vi "Main.vi"(11 "Module Admin":refnum<class "Delacor_lib_QMH_Module Admin.lvclass">) -> ()   [LabVIEW 2019, in "Acquisition.lvlib"]
doc: "This template is based off of the Queued Message Handler design pattern and the Queued Message Handler project template that ships with LabVIEW.\n\nThe main difference is that the queue is private to this module and communication between modules is performed via Broadcast and Request events.\n\nRequest events are wrapped in public API methods and are handled in the Event Handling Loop (EHL) of this VI. Any module can register for Broadcast events sent by this module. The EHL generates messages based on user interface actions.\n\nThe Message Handling Loop (MHL) processes messages generated by the EHL, or by other messages. The messages are string values, so new messages can be added easily to the Message Cases case structure in the MHL. Each message cluster can also provide an optional value for Message Data, which is a variant that can be converted to whatever message-specific data is required.\n_____\nBased on Delacor QMH Project Template 4.0.0.47.\n_____\nBased on Delacor QMH Project Template 5.0.0.82."
uses:
  Acquisition.lvlib
  <vilib>/Delacor/Delacor QMH/Libraries/Module Admin_class/Delacor_lib_QMH_Module Admin.lvclass
  Module Data--cluster.ctl
  Stop Argument--cluster.ctl
  <vilib>/Delacor/Delacor QMH/Libraries/Message Queue_class/Delacor_lib_QMH_Message Queue.lvclass/Delacor_lib_QMH_Message Queue.ctl
  <vilib>/Delacor/Delacor QMH/Libraries/Module Admin_class/Delacor_lib_QMH_Module Admin.lvclass/Delacor_lib_QMH_Module Admin.ctl
  Start Acquiring Argument--cluster.ctl
  Start Acquiring (Reply Payload)--cluster.ctl
  Stop Acquiring Argument--cluster.ctl
  Settings Editor/Update Application Settings (Reply Payload)--cluster.ctl
  Settings Editor/Settings--cluster.ctl
  <vilib>/Utility/miscctls.llb/LVPointTypeDef.ctl
  <vilib>/Delacor/Delacor QMH/Libraries/Message Queue_class/Delacor_lib_QMH_Enqueue Message (Single).vi
  <vilib>/Delacor/Delacor QMH/Libraries/Module Admin_class/Delacor_lib_QMH_Get External Launch.vi
  <vilib>/Utility/error.llb/Error Cluster From Error Code.vi
  <vilib>/ErrorRing/Error Ring.xnode
  <vilib>/Delacor/Delacor QMH/Libraries/Message Queue_class/Delacor_lib_QMH_Message Queue.lvclass
  Settings Editor/Settings Editor.lvlib
  Logger/Logger.lvlib
panel:
  out "Settings":T1={"Analog Input Channel"="", "Max Value"=0.0, "Min Value"=-5.0}
  out "Graph Data":waveform(dbl)[](array[waveform])
  out "error out":errorcluster
  # "This is a headless module. Show its panel to confirm that the Settings are updated correctly and other debugging tasks. Use the Settings Editor to change the settings for this module."
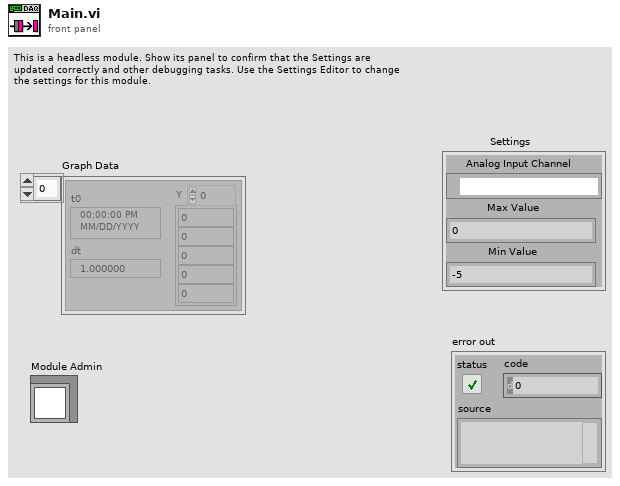
[diagram p1: front panel]
types:
  T1 = typedef "Acquisition.lvlib/Module Data--cluster.ctl" = cluster{"Analog Input Channel":refnum<k21>, "Max Value":dbl, "Min Value":dbl}
  T2 = typedef "Settings Editor.lvlib/Broadcast Events--cluster.ctl" = cluster{"Module Did Init":refnum<user-event>, "Status Updated":refnum<user-event>, "Error Reported":refnum<user-event>, "Module Did Stop":refnum<user-event>, "Update Module Execution Status":refnum<user-event>, "Application Settings Updated":refnum<user-event>}
  T3 = typedef "Acquisition.lvlib/Request Events--cluster.ctl" = cluster{"Stop Module":refnum<user-event>, "Show Panel":refnum<user-event>, "Hide Panel":refnum<user-event>, "Get Module Execution Status":refnum<user-event>, "Show Diagram":refnum<user-event>, "Stop Acquiring":refnum<user-event>, "Wakeup Helper Loop":refnum<user-event>, "Change Settings":refnum<user-event>, "Calibrate DAQ":refnum<user-event>, "Start Acquiring":refnum<user-event>}
  T4 = enum32{"invalid lock state", "Not Locked", "Locked (No Password)", "Password-protected"}
  T5 = typedef "Acquisition.lvlib/Stop Argument--cluster.ctl" = cluster{"Origin":string, "Exit via Stop Module Req?":bool, "Wait for Module to stop?":bool}
  T6 = typedef "Acquisition.lvlib/Start Acquiring Argument--cluster.ctl" = cluster{"Wait Notifier":refnum<notifier>, "wait for reply":bool}
  T7 = typedef "Acquisition.lvlib/Stop Acquiring Argument--cluster.ctl" = cluster{"Boolean":bool}
  T8 = typedef "Settings Editor.lvlib/Update Application Settings (Reply Payload)--cluster.ctl" = cluster{"Settings":T9, "Update Settings_error":errorcluster}
  T9 = typedef "Settings Editor.lvlib/Settings--cluster.ctl" = cluster{"Log File Base Path":path, "Analog Input Channel":refnum<k21>, "Max Value":dbl, "Min Value":dbl}
  T10 = typedef "LVPointTypeDef.ctl" = cluster{"Horizontal":i16, "Vertical":i16}
  T11 = enum32{"Invalid", "Standard", "Closed", "Hidden", "Minimized", "Maximized"}
  T12 = typedef "Acquisition.lvlib/Start Acquiring (Reply Payload)--cluster.ctl" = cluster{"HW ID":string, "Start Acquiring_error":errorcluster}
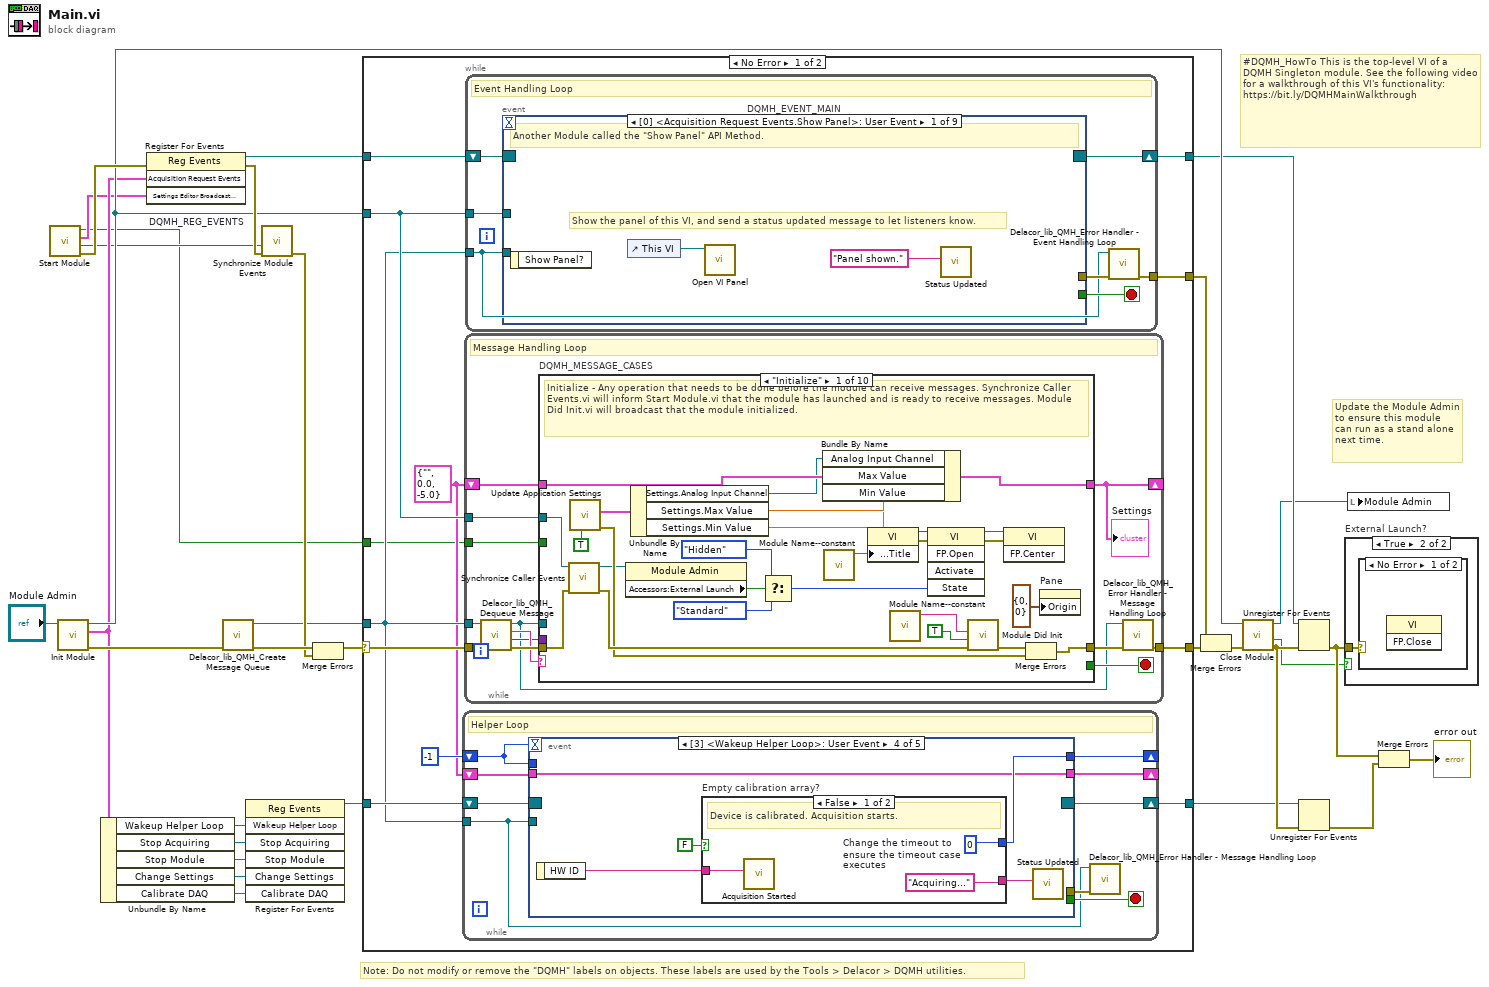
[diagram p0: block diagram]
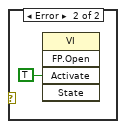
[diagram p3: hidden frame]
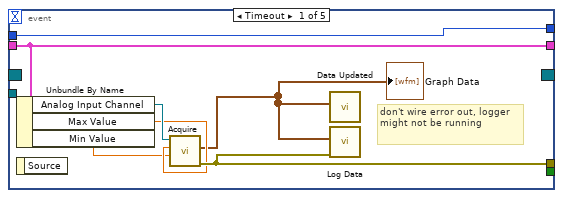
[diagram p4: hidden frame]
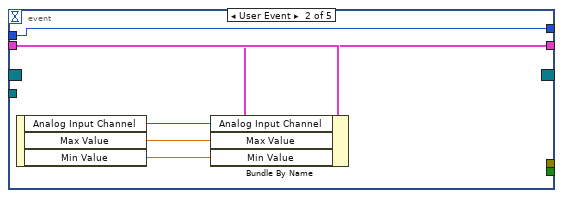
[diagram p5: hidden frame]
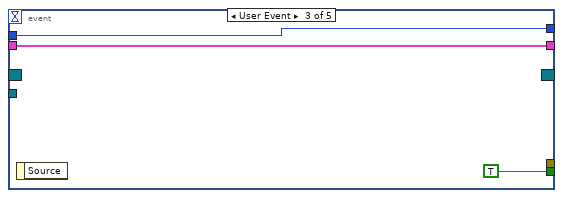
[diagram p6: hidden frame]
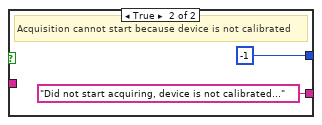
[diagram p7: hidden frame]
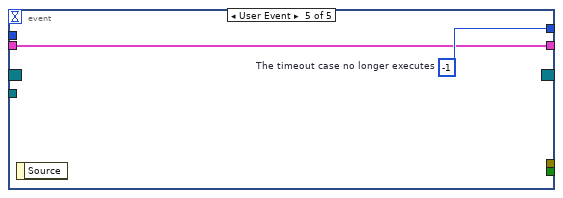
[diagram p8: hidden frame]
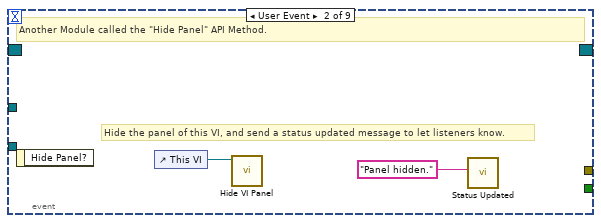
[diagram p9: hidden frame]
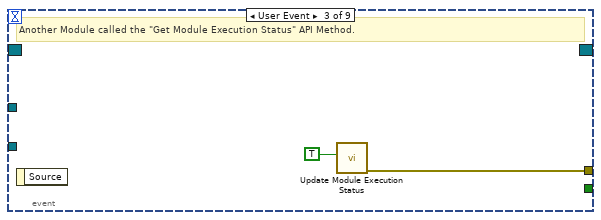
[diagram p10: hidden frame]
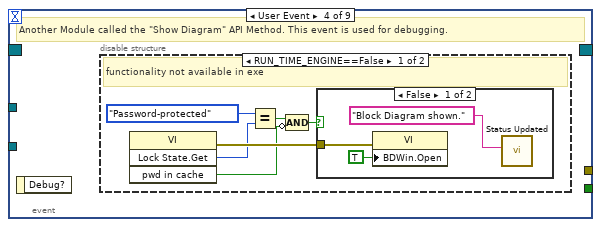
[diagram p11: hidden frame]
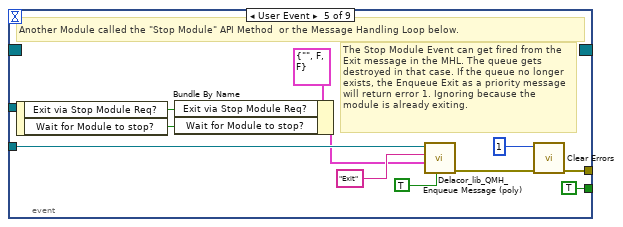
[diagram p14: hidden frame]
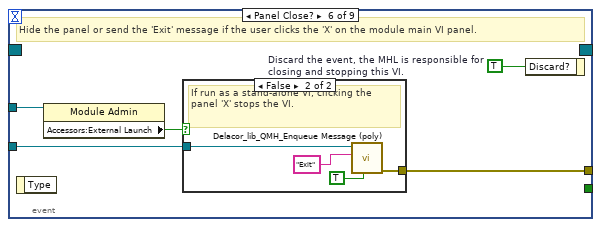
[diagram p15: hidden frame]
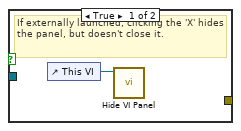
[diagram p16: hidden frame]
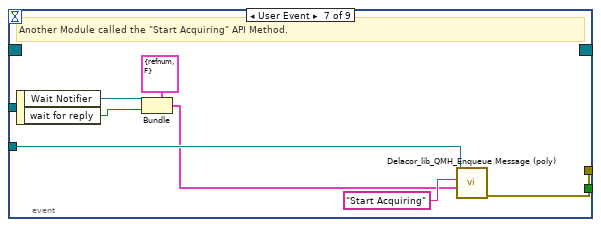
[diagram p17: hidden frame]
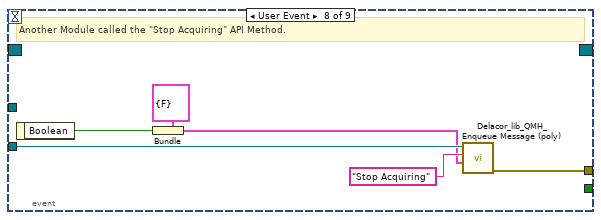
[diagram p18: hidden frame]
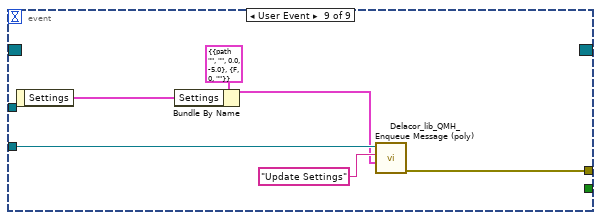
[diagram p19: hidden frame]
diagram:
  # "#DQMH_HowTo This is the top-level VI of a DQMH Singleton module. See the following video for a walkthrough of this VI's functionality: https://bit.ly/DQMHMainWalkthrough"
  # "Note: Do not modify or remove the \"DQMH\" labels on objects. These labels are used by the Tools > Delacor > DQMH utilities."
  # "Update the Module Admin to ensure this module can run as a stand alone next time."
  n1 = call "Start Module.vi"() -> ("error out"=w24:errorcluster, "Wait for Event Sync?"=w5:bool, "Settings Editor Broadcast Events"=w6:T2, "Module Was Already Running?"=w1:bool)  [unwired: 8 in]
  n2 = call "Init Module.vi"("Singleton Module Admin in"="Module Admin") -> ("error out"=w30:errorcluster, "Acquisition Request Events"=w11:T3, "Singleton Module Admin out"=w18:refnum<class "Delacor_lib_QMH_Module Admin.lvclass">)  [unwired: 8 in]
  n3 = Unbundle By Name(w11) -> ("Wakeup Helper Loop"=w7:refnum<user-event>, "Stop Acquiring"=w10:refnum<user-event>, "Stop Module"=w9:refnum<user-event>, "Change Settings"=w4:refnum<user-event>, "Calibrate DAQ"=w3:refnum<user-event>)
  n4 = register-events "DQMH_REG_EVENTS"(error in=w24, w11, w6) -> (reference out=w16:refnum<event-registration>, error out=w23:errorcluster)  [unwired: 1 in]
  n5 = call <vilib>:"Delacor_lib_QMH_Create Message Queue.vi"("error in"=w30) -> ("error out"=w26:errorcluster, "Message Queue"=w15:refnum<class "Delacor_lib_QMH_Message Queue.lvclass">)  [unwired: 9 in]
  n6 = register-events(w7, w10, w9, w4, w3) -> (reference out=w8:refnum<event-registration>)  [unwired: 2 in, 1 out]
  n7 = call "Synchronize Module Events.vi"("error in (no error)"=w23, "Wait for Event Sync?"=w5) -> ("error out"=w22:errorcluster)  [unwired: 9 in]
  n8 = Merge Errors(w26, w22) -> (w25:errorcluster)
  n9 = case shown="No Error" w25 {
    selector: w25 -> [w41 w279]
    tunnel: [w43 w278] -> w31
    tunnel: [w40 w287] -> w17
    tunnel: w16 -> [w39 w287]
    tunnel: w15 -> [w35 w280]
    tunnel: [w42 _] -> w29
    tunnel: w18 -> [w38 w283]
    tunnel: w8 -> [w36 w282]
    tunnel: [w33 w282] -> w2
    tunnel: w1 -> [w32 w281]
    frame No Error {
      w34 = T1 {"Analog Input Channel"="", "Max Value"=0.0, "Min Value"=-5.0} ("Data Cluster")
      n10 = while {
        shift-right: [w51] -> _
        shift-left: -1 -> [w50]
        tunnel: w35 -> [w47]
        shift-right: [w46] -> _
        shift-left: w34 -> [w45]
        shift-right: [w44] -> w33
        shift-left: w36 -> [w49]
        stop <- w48 stop-if-true
        # "Helper Loop"
        n11 = event shown="[3] <Wakeup Helper Loop>: User Event" {
          selector: w49 -> [_ _ _ _ _]
          dyn-events: [_ _ _ _ _] -> w44
          timeout: w50 -> [_ _ _ _ _]
          tunnel: [w58 w65 w68 w73 w80] -> w51
          tunnel: w50 -> [w58 w65 w68 _ _]
          tunnel: [_ _ TRUE _ _] -> w48
          tunnel: w47 -> [_ _ _ _ _]
          tunnel: [w59 _ _ _ _] -> w52
          tunnel: [w57 w63 w66 w70 w79] -> w46
          tunnel: w45 -> [w57 w64 w66 w70 w79]
          event Timeout {
            # "don't wire error out, logger might not be running"
            n12 = Unbundle By Name(w57) -> ("Analog Input Channel"=w56:refnum<k21>, "Max Value"=w55:dbl, "Min Value"=w54:dbl)
            n13 = event-data() -> ()  [unwired: 1 in, 1 out]
            n14 = call "Acquire.vi"("Min Value"=w54, "Max Value"=w55, "Refnum in"=w56) -> ("error out"=w59:errorcluster, "Graph Data"=w53:waveform(dbl)[])  [unwired: 7 in]
            "Graph Data" <- w53
            n15 = call "Data Updated.vi"("Graph Data"=w53) -> ()  [unwired: 10 in, 1 out]
            n16 = call "Log Data.vi"("error in (no error)"=w59, "Waveforms"=w53) -> ()  [unwired: 9 in, 1 out]
          }
          event User Event {
            n17 = event-data() -> ("Analog Input Channel"=w60:refnum<k21>, "Max Value"=w62:dbl, "Min Value"=w61:dbl)  [unwired: 1 in]
            n18 = Bundle By Name(cluster=w64, "Analog Input Channel"=w60, "Max Value"=w62, "Min Value"=w61) -> (w63:T1)
          }
          event User Event {
            n19 = event-data() -> ()  [unwired: 1 in, 1 out]
          }
          event User Event {
            n20 = event-data() -> ("HW ID"=w71:string)  [unwired: 1 in]
            n21 = case "Empty calibration array?" shown="False" FALSE {
              tunnel: ["Acquiring..." ("Status") "Did not start acquiring, device is not calibrated..." ("Status")] -> w72
              tunnel: [w75 -1] -> w73
              tunnel: w71 -> [w76 _]
              frame False {
                w75 = 0  # Change the timeout to ensure the timeout case executes
                # "Device is calibrated. Acquisition starts."
                n22 = call "Acquisition Started.vi"("HW ID"=w76) -> ()  [unwired: 10 in, 1 out]
              }
              frame True {
                # "Acquisition cannot start because device is not calibrated"
              }
            }
            n23 = call "Status Updated.vi"("Status"=w72) -> ()  [unwired: 10 in, 1 out]
          }
          event User Event {
            w80 = -1  # The timeout case no longer executes
            n24 = event-data() -> ()  [unwired: 1 in, 1 out]
          }
        }
        n25 = call-dynamic "Delacor_lib_QMH_Error Handler - Message Handling Loop.vi"("error in"=w52, "Message Queue in"=w47) -> ()  [unwired: 8 in, 2 out]
      }
      n26 = while {
        tunnel: w35 -> [w147]
        shift-right: [w143] -> _
        shift-left: w34 -> [w151]
        tunnel: w41 -> [w154]
        tunnel: [w152] -> w43
        tunnel: w38 -> [w145]
        tunnel: w32 -> [w144]
        stop <- w150 stop-if-true
        # "Message Handling Loop"
        n27 = call-dynamic "Delacor_lib_QMH_Dequeue Message.vi"("error in"=w154, "Message Queue in"=w147) -> ("error out"=w153:errorcluster, "Message Data"=w148:variant, "Message"=w149:string, "Message Queue out"=w146:refnum<class "Delacor_lib_QMH_Message Queue.lvclass">)  [unwired: 6 in]
        n28 = case "DQMH_MESSAGE_CASES" shown="\"Initialize\"" w149 {
          selector: w149 -> [_ _ _ _ _ _ _ _ _ w265]
          tunnel: w146 -> [_ _ _ _ _ _ _ w230 w254 _]
          tunnel: w153 -> [w179 w183 w196 w210 w221 w224 w226 w237 w261 w268]
          tunnel: [w176 w183 w194 w208 w213 w223 w226 w233 w258 w269] -> w155
          tunnel: w151 -> [w166 w182 w184 w205 w218 w222 w225 w232 w246 w266]
          tunnel: [w161 w182 w192 w205 w218 w222 w225 w232 w246 w266] -> w143
          tunnel: [_ _ _ _ _ _ _ _ w253 _] -> w150
          tunnel: w148 -> [_ _ w191 w207 w219 _ _ w231 w252 _]
          tunnel: w145 -> [w167 _ _ _ _ _ _ w229 w247 _]
          tunnel: w144 -> [_ _ _ _ _ _ _ _ w244 _]
          frame "Initialize" {
            # "Initialize - Any operation that needs to be done before the module can receive messages. Synchronize Caller Events.vi will inform Start Module.vi that the module has launched and is ready to receive messages. Module Did Init.vi will broadcast that the module initialized."
            n29 = call "Synchronize Caller Events.vi"("error in (no error)"=w179, "Singleton Module Admin in"=w167) -> ("error out"=w178:errorcluster, "Singleton Module Admin out"=w163:refnum<class "Delacor_lib_QMH_Module Admin.lvclass">)  [unwired: 8 in]
            n30 = call "Update Application Settings.vi"("wait for reply (T)"=TRUE) -> ("error out"=w175:errorcluster, "Reply Payload"=w160:T8)  [unwired: 8 in, 1 out]
            n31 = property class="Module Admin"(reference=w163) -> ("Accessors:External Launch"=w171:bool)  [unwired: 1 in, 2 out]
            n32 = Unbundle By Name(w160) -> ("Settings.Analog Input Channel"=w156:refnum<k21>, "Settings.Max Value"=w159:dbl, "Settings.Min Value"=w158:dbl)
            n33 = Select(t=T11."Hidden" ("State"), s=w171, f=T11."Standard" ("State")) -> (s? t:f=w168:T11)
            n34 = Bundle By Name(cluster=w166, "Analog Input Channel"=w156, "Max Value"=w159, "Min Value"=w158) -> (w161:T1)
            n35 = call "Module Name--constant.vi"() -> ("Module Name"=w174:string)  [unwired: 11 in]
            n36 = property class="VI"("Front Panel.Title"=w174) -> (reference out=w173:refnum<vi>, error out=w181:errorcluster)  [unwired: 2 in]
            n37 = call "Module Name--constant.vi"() -> ("Module Name"=w164:string)  [unwired: 11 in]
            n38 = invoke class="VI" method="FP.Open"(reference=w173, error in=w181, "State"=w168) -> (reference out=w172:refnum<vi>, error out=w180:errorcluster)  [unwired: 2 in, 3 out]
            n39 = call "Module Did Init.vi"("error in (no error)"=w178, "Initialized?"=TRUE, "Origin"=w164) -> ("error out"=w177:errorcluster)  [unwired: 8 in]
            n40 = invoke class="VI" method="FP.Center"(reference=w172, error in=w180) -> ()  [unwired: 1 in, 3 out]
            n41 = Merge Errors(w177, w175) -> (w176:errorcluster)
            n42 = property on="Pane" class="Pane"("Origin"=T10 {"Horizontal"=0, "Vertical"=0}) -> ()  [unwired: 2 in, 2 out]
          }
          frame "--- Module Specific ---" {
            # "Separator -- The following cases handle messages specific to this Module."
          }
          frame "Start Acquiring" {
            # "Requests Acquisition Module to start acquiring."
            n43 = Variant To Data(error in=w196, type=T6 {"Wait Notifier"=refnum, "wait for reply"=FALSE} ("Start Acquisition Argument"), Variant=w191) -> (data=w189:T6, error out=w193:errorcluster)
            n44 = in-place {
              in-place-border: [w202] -> w195
              in-place-border: w193 -> [w201]
              in-place-border: [w197] -> w185
              n45 = in-place-cluster #1(w184) -> ("Analog Input Channel"=w198:refnum<k21>)
              n46 = call "Initialize Hardware References.vi"("error in (no error)"=w201, "HW Refnum in"=w198) -> ("error out"=w200:errorcluster, "HW Refnum out"=w199:string)  [unwired: 8 in]
              n47 = call "Configure Hardware.vi"("error in (no error)"=w200, "HW Refnum in"=w199) -> ("error out"=w202:errorcluster, "HW Refnum out"=w197:string)  [unwired: 8 in]
              n48 = in-place-cluster #1("Analog Input Channel"=w197) -> (w192:T1)
            }
            n49 = Bundle By Name(cluster=T12 {"HW ID"="", "Start Acquiring_error"={"status"=FALSE, "code"=0, "source"=""}} ("Start Acquisition (Reply Payload)"), "HW ID"=w185, "Start Acquiring_error"=w195) -> (w187:T12)
            n50 = Unbundle By Name(w189) -> ("Wait Notifier"=w188:refnum<notifier>)
            n51 = call "Wakeup Helper Loop.vi"("error in (no error)"=w195, "HW ID"=w185) -> ("error out"=w194:errorcluster)  [unwired: 9 in]
            n52 = Send Notification(notification=w187, notifier=w188) -> ()  [unwired: 1 in, 2 out]
          }
          frame "Stop Acquiring" {
            # "Requests the Acquisition Module to stop acquiring"
            n53 = Variant To Data(error in=w210, type=T7 {"Boolean"=FALSE} ("Stop Acquiring Argument"), Variant=w207) -> (error out=w209:errorcluster)  [unwired: 1 out]
            n54 = Unbundle By Name(w205) -> ("Analog Input Channel"=w204:refnum<k21>)
            n55 = call "Stop Acquisition.vi"("error in (no error)"=w209, "HW Refnum"=w204) -> ("error out"=w208:errorcluster)  [unwired: 9 in]
            n56 = call "Acquisition Stopped.vi"("error in (no error)"=w208) -> ()  [unwired: 10 in, 1 out]
            n57 = call "Status Updated.vi"("error in (no error)"=w208, "Status"="Acquisition Stopped") -> ()  [unwired: 9 in, 1 out]
          }
          frame "Update Settings" {
            # "Send the Change Settings event to the helper loop."
            # "The Settings Editor broadcasted that the settings have changed."
            n58 = Variant To Data(error in=w221, type=T8 {"Settings"={"Log File Base Path"=path "", "Analog Input Channel"="", "Max Value"=0.0, "Min Value"=-5.0}, "Update Settings_error"={"status"=FALSE, "code"=0, "source"=""}} ("Settings Updated Argument"), Variant=w219) -> (data=w216:T8, error out=w220:errorcluster)
            n59 = Unbundle By Name(w216) -> ("Settings.Analog Input Channel"=w211:refnum<k21>, "Settings.Max Value"=w215:dbl, "Settings.Min Value"=w214:dbl)
            n60 = call "Change Settings.vi"("error in (no error)"=w220, "Min Value"=w214, "Max Value"=w215, "Analog Input Channel"=w211) -> ("error out"=w213:errorcluster)  [unwired: 7 in]
            n61 = call "Status Updated.vi"("error in (no error)"=w213, "Status"="Settings Updated") -> ()  [unwired: 9 in, 1 out]
          }
          frame "---Copy This Frame---" {
            # "Duplicate this frame when creating new messages.  Change this comment in the duplicated frame to describe this message."
            n62 = Merge Errors(w224) -> (w223:errorcluster)
          }
          frame "--- Exit and Error Handling---" {
            # "Separator - The following cases handle errors and exit messages."
          }
          frame "Error" {
            # "Error - Check the error message data and respond accordingly. This message is sent by the \"Error Handler\" VIs at the end of each loop in this application."
            n63 = property class="Module Admin"(reference=w229) -> ("Accessors:External Launch"=w228:bool)  [unwired: 1 in, 2 out]
            n64 = Variant To Data(error in=w237, type=errorcluster {"status"=FALSE, "code"=0, "source"=""} ("error constant"), Variant=w231) -> (data=w238:errorcluster, error out=w235:errorcluster)
            n65 = call "Module Name--constant.vi"() -> ("Module Name"=w227:string)  [unwired: 11 in]
            n66 = call "Error Reported.vi"("Additional Information"=w227, "Error"=w238) -> ()  [unwired: 9 in, 1 out]
            n67 = case shown="False" w228 {
              tunnel: [w243 _] -> w234
              tunnel: w230 -> [w241 _]
              tunnel: w238 -> [w242 _]
              frame False {
                # "If the module is running standalone, then pop up an error dialog and call the \"Exit\" message."
                n68 = call <vilib>:"Simple Error Handler.vi"("error in (no error)"=w242) -> ()  [unwired: 4 in, 5 out]
                n69 = call-poly <vilib>:"Delacor_lib_QMH_Enqueue Message (poly).vi"("Priority Message? (F)"=TRUE, "Message"="Exit", "Message Queue in"=w241) -> ("error out"=w243:errorcluster)  [unwired: 7 in, 1 out]
              }
              frame True {
                # "If the module was launched externally, calling the Error Reported broadcast VI is the only action performed by the \"Error\" message. The module's caller can then process the error appropriately."
              }
            }
            n70 = Merge Errors(w235, w234) -> (w233:errorcluster)
            n71 = local write "error out"(w233) -> ()
          }
          frame "Exit" {
            w251 = 91  # 91: not all Exit messages will have an argument
            w253 = TRUE  # Stop the VI
            # "Release the message queue reference"
            # "Exit - Exit the application."
            n72 = Variant To Data(error in=w261, type=T5 {"Origin"="", "Exit via Stop Module Req?"=FALSE, "Wait for Module to stop?"=FALSE} ("Stop Argument"), Variant=w252) -> (data=w249:T5, error out=w257:errorcluster)
            n73 = call <vilib>:"Clear Errors.vi"("error in (no error)"=w257, "specific error code to clear (0: all)"=w251) -> ("error out"=w260:errorcluster)  [unwired: 4 in, 1 out]
            n74 = Unbundle By Name(w246) -> ("Analog Input Channel"=w245:refnum<k21>)
            n75 = control-ref of="This VI"() -> (w248:refnum<vi>)
            n76 = call "Handle Exit.vi"("Stop Argument"=w249, "Admin in"=w247, "VI reference"=w248) -> ("error out"=w256:errorcluster)  [unwired: 7 in, 1 out]
            n77 = call "Close Hardware References.vi"("HW Refnum in"=w245) -> ("error out"=w255:errorcluster)  [unwired: 9 in, 1 out]
            n78 = call-dynamic "Delacor_lib_QMH_Release Message Queue.vi"("error in"=w260, "Message Queue"=w254) -> ("error out"=w259:errorcluster)  [unwired: 9 in]
            n79 = case "Settings Editor was\nalready running?" shown="False" w244 {
              frame False {
                n80 = call "Module Name--constant.vi"() -> ("Module Name"=w263:string)  [unwired: 11 in]
                n81 = call "Stop Module.vi"("Wait for Module to Stop? (F)"=TRUE, "Origin"=w263) -> ()  [unwired: 9 in, 1 out]
              }
              frame True {
                # "Another Module is\nin charge of stopping Settings Editor"
              }
            }
            n82 = Merge Errors(w259, w256, w255) -> (w258:errorcluster)
          }
          frame Default {
            # "'Default' case only runs if there is a message that isn't defined in any of the other cases.  Output a programming error."
            n83 = call "Module Name--constant.vi"() -> ("Module Name"=w264:string)  [unwired: 11 in]
            n84 = xnode "Error Ring"("parameter 0"=w265, "parameter 1"=w264) -> ("error out"=w267:errorcluster)
            n85 = Merge Errors(w268, w267) -> (w269:errorcluster)
          }
        }
        "Settings" <- w143
        n86 = call-dynamic "Delacor_lib_QMH_Error Handler - Message Handling Loop.vi"("error in"=w155, "Message Queue in"=w146) -> ("dup error in"=w152:errorcluster)  [unwired: 8 in, 1 out]
      }
      n87 = while {
        tunnel: w35 -> [w81]
        shift-right: [w84] -> w40
        shift-left: w39 -> [w85]
        tunnel: [w86] -> w42
        tunnel: w38 -> [w82]
        stop <- w83 stop-if-true
        # "Event Handling Loop"
        n88 = event "DQMH_EVENT_MAIN" shown="[0] <Acquisition Request Events.Show Panel>: User Event" {
          selector: w85 -> [_ _ _ _ _ _ _ _ _]
          dyn-events: [_ _ _ _ _ _ _ _ _] -> w84
          timeout: _ -> [_ _ _ _ _ _ _ _ _]
          tunnel: [_ _ _ _ TRUE ("Discard?") _ _ _ _] -> w83
          tunnel: w81 -> [_ _ _ _ w109 w116 w130 w135 w140]
          tunnel: [_ _ w93 _ w112 w118 w126 w136 w142] -> w87
          tunnel: w82 -> [_ _ _ _ _ w115 _ _ _]
          event User Event {
            # "Show the panel of this VI, and send a status updated message to let listeners know."
            # "Another Module called the \"Show Panel\" API Method."
            n89 = event-data() -> ()  [unwired: 1 in, 1 out]
            n90 = control-ref of="This VI"() -> (w89:refnum<vi>)
            n91 = call "Open VI Panel.vi"("VI"=w89) -> ()  [unwired: 10 in, 1 out]
            n92 = call "Status Updated.vi"("Status"="Panel shown." ("format string")) -> ()  [unwired: 10 in, 1 out]
          }
          event User Event {
            # "Hide the panel of this VI, and send a status updated message to let listeners know."
            # "Another Module called the \"Hide Panel\" API Method."
            n93 = event-data() -> ()  [unwired: 1 in, 1 out]
            n94 = control-ref of="This VI"() -> (w91:refnum<vi>)
            n95 = call "Hide VI Panel.vi"("VI"=w91) -> ()  [unwired: 10 in, 1 out]
            n96 = call "Status Updated.vi"("Status"="Panel hidden." ("format string")) -> ()  [unwired: 10 in, 1 out]
          }
          event User Event {
            # "Another Module called the \"Get Module Execution Status\" API Method."
            n97 = event-data() -> ()  [unwired: 1 in, 1 out]
            n98 = call "Update Module Execution Status.vi"("Running?"=TRUE) -> ("error out"=w93:errorcluster)  [unwired: 10 in]
          }
          event User Event {
            # "Another Module called the \"Show Diagram\" API Method. This event is used for debugging."
            n99 = event-data() -> ()  [unwired: 1 in, 1 out]
            n100 = disable-structure shown="RUN_TIME_ENGINE==False" {
              frame condition #0 (active) {
                # "functionality not available in exe"
                n101 = invoke class="VI" method="Lock State.Get"() -> (error out=w99:errorcluster, "Get Lock State"=w98:T4, "pwd in cache"=w95:bool)  [unwired: 4 in, 1 out]
                n102 = Equal?(x=T4."Password-protected", y=w98) -> (x = y?=w96:bool)
                n103 = Compound Arithmetic op=AND(w96, invert w95) -> (w94:bool)
                n104 = case shown="False" w94 {
                  tunnel: w99 -> [w102 _]
                  frame False {
                    n105 = property class="VI"(error in=w102, "BDWin.Open"=TRUE ("Block Diagram Window:Open")) -> ()  [unwired: 1 in, 2 out]
                    n106 = call "Status Updated.vi"("Status"="Block Diagram shown." ("format string")) -> ()  [unwired: 10 in, 1 out]
                  }
                  frame True {
                    # "Password-protected VI, and the password is not in the cache. Do not show the diagram."
                  }
                }
              }
              frame condition #1 {
              }
            }
          }
          event User Event {
            # "The Stop Module Event can get fired from the Exit message in the MHL. The queue gets destroyed in that case. If the queue no longer exists, the Enqueue Exit as a priority message will return error 1. Ignoring because the module is already exiting."
            # "Another Module called the \"Stop Module\" API Method  or the Message Handling Loop below."
            n107 = event-data() -> ("Exit via Stop Module Req?"=w105:bool, "Wait for Module to stop?"=w104:bool)  [unwired: 1 in]
            n108 = Bundle By Name(cluster=T5 {"Origin"="", "Exit via Stop Module Req?"=FALSE, "Wait for Module to stop?"=FALSE} ("Stop Argument"), "Exit via Stop Module Req?"=w105, "Wait for Module to stop?"=w104) -> (w103:T5)
            n109 = call-poly <vilib>:"Delacor_lib_QMH_Enqueue Message (poly).vi"("Priority Message? (F)"=TRUE, "Message Data"=w103, "Message"="Exit", "Message Queue in"=w109) -> ("error out"=w113:errorcluster)  [unwired: 6 in, 1 out]
            n110 = call <vilib>:"Clear Errors.vi"("error in (no error)"=w113, "specific error code to clear (0: all)"=1) -> ("error out"=w112:errorcluster)  [unwired: 4 in, 1 out]
          }
          event Panel Close? {
            w117 = TRUE  # Discard the event, the MHL is responsible for closing and stopping this VI.
            # "Hide the panel or send the 'Exit' message if the user clicks the 'X' on the module main VI panel."
            n111 = event-data() -> ()  [unwired: 1 in, 1 out]
            n112 = property class="Module Admin"(reference=w115) -> ("Accessors:External Launch"=w114:bool)  [unwired: 1 in, 2 out]
            n113 = case shown="False" w114 {
              tunnel: w116 -> [_ w122]
              tunnel: [_ w123] -> w118
              frame True {
                # "If externally launched, clicking the 'X' hides the panel, but doesn't close it."
                n114 = control-ref of="This VI"() -> (w119:refnum<vi>)
                n115 = call "Hide VI Panel.vi"("VI"=w119) -> ()  [unwired: 10 in, 1 out]
              }
              frame False {
                # "If run as a stand-alone VI, clicking the panel 'X' stops the VI."
                n116 = call-poly <vilib>:"Delacor_lib_QMH_Enqueue Message (poly).vi"("Priority Message? (F)"=TRUE, "Message"="Exit", "Message Queue in"=w122) -> ("error out"=w123:errorcluster)  [unwired: 7 in, 1 out]
              }
            }
            n117 = event-data("Discard?"=w117) -> ()  [unwired: 1 in, 1 out]
          }
          event User Event {
            # "Another Module called the \"Start Acquiring\" API Method."
            n118 = event-data() -> ("Wait Notifier"=w125:refnum<notifier>, "wait for reply"=w124:bool)  [unwired: 1 in]
            n119 = Bundle(cluster=T6 {"Wait Notifier"=refnum, "wait for reply"=FALSE} ("Start Acquisition Argument"), "Wait Notifier"=w125, "wait for reply"=w124) -> (w127:T6)
            n120 = call-poly <vilib>:"Delacor_lib_QMH_Enqueue Message (poly).vi"("Message Data"=w127, "Message"="Start Acquiring", "Message Queue in"=w130) -> ("error out"=w126:errorcluster)  [unwired: 7 in, 1 out]
          }
          event User Event {
            # "Another Module called the \"Stop Acquiring\" API Method."
            n121 = event-data() -> ("Boolean"=w131:bool)  [unwired: 1 in]
            n122 = Bundle(cluster=T7 {"Boolean"=FALSE} ("Stop Acquiring Argument"), "Boolean"=w131) -> (w132:T7)
            n123 = call-poly <vilib>:"Delacor_lib_QMH_Enqueue Message (poly).vi"("Message Data"=w132, "Message"="Stop Acquiring", "Message Queue in"=w135) -> ("error out"=w136:errorcluster)  [unwired: 7 in, 1 out]
          }
          event User Event {
            n124 = event-data() -> ("Settings"=w137:T9)  [unwired: 1 in]
            n125 = Bundle By Name(cluster=T8 {"Settings"={"Log File Base Path"=path "", "Analog Input Channel"="", "Max Value"=0.0, "Min Value"=-5.0}, "Update Settings_error"={"status"=FALSE, "code"=0, "source"=""}} ("Settings Updated Argument"), "Settings"=w137) -> (w139:T8)
            n126 = call-poly <vilib>:"Delacor_lib_QMH_Enqueue Message (poly).vi"("Message Data"=w139, "Message"="Update Settings", "Message Queue in"=w140) -> ("error out"=w142:errorcluster)  [unwired: 7 in, 1 out]
          }
        }
        n127 = call-dynamic "Delacor_lib_QMH_Error Handler - Event Handling Loop.vi"("error in"=w87, "Message Queue in"=w81) -> ("dup error in"=w86:errorcluster)  [unwired: 8 in, 1 out]
      }
    }
    frame Error {
      # "Synchronize Caller Events.vi will inform Start Module.vi that the module has launched and will let the code calling Start Module.vi register for broadcasts and would permit the caller receive the broadcast that an error occurred at launch time."
      n128 = call "Synchronize Caller Events.vi"("Singleton Module Admin in"=w283) -> ("error out"=w288:errorcluster)  [unwired: 9 in, 1 out]
      n129 = call-dynamic "Delacor_lib_QMH_Release Message Queue.vi"("error in"=w279, "Message Queue"=w280) -> ("error out"=w278:errorcluster)  [unwired: 9 in]
      n130 = call "Module Name--constant.vi"() -> ("Module Name"=w286:string)  [unwired: 11 in]
      n131 = case "Settings Editor was\nalready running?" shown="False" w281 {
        frame False {
          n132 = call "Module Name--constant.vi"() -> ("Module Name"=w291:string)  [unwired: 11 in]
          n133 = call "Stop Module.vi"("Wait for Module to Stop? (F)"=TRUE, "Origin"=w291) -> ()  [unwired: 9 in, 1 out]
        }
        frame True {
          # "Another Module is\nin charge of stopping Settings Editor"
        }
      }
      n134 = Format Into String(format string="An error occurred during initialization. %s is no longer running.", w286) -> (resulting string=w284:string)  [unwired: 2 in, 1 out]
      n135 = Merge Errors(w278, w288) -> (w289:errorcluster)
      n136 = call "Error Reported.vi"("Additional Information"=w284, "Error"=w289) -> ()  [unwired: 9 in, 1 out]
    }
  }
  n137 = Merge Errors(w29, w31) -> (w28:errorcluster)
  n138 = call "Close Module.vi"("error in (no error)"=w28, "Module Admin in"=w18) -> ("error out"=w21:errorcluster, "External Launch"=w12:bool, "Module Admin out"=w13:refnum<class "Delacor_lib_QMH_Module Admin.lvclass">)  [unwired: 7 in]
  n139 = Unregister For Events(event registration refnum=w17, error in=w21) -> (error out=w27:errorcluster)
  n140 = Unregister For Events(event registration refnum=w2, error in=w21) -> (error out=w19:errorcluster)
  n141 = case "External Launch?" shown="True" w12 {
    tunnel: w27 -> [_ w292]
    frame False {
    }
    frame True {
      n142 = case shown="No Error" w292 {
        frame No Error {
          n143 = invoke class="VI" method="FP.Close"() -> ()  [unwired: 3 in, 3 out]
        }
        frame Error {
          n144 = invoke class="VI" method="FP.Open"("Activate"=TRUE ("Activate?")) -> ()  [unwired: 4 in, 5 out]
        }
      }
    }
  }
  n145 = local write "Module Admin"(w13) -> ()
  n146 = Merge Errors(w27, w19) -> (→"error out":errorcluster)
